vi "connectAndReceiveMessages.vi"(8 "error in (no error)":errorcluster, 9 "remote port":u16, 10 "remote address":string, 11 "NetworkServer in":refnum<class "NetworkServer.lvclass">) -> (0 "error out":errorcluster, 3 "NetworkServer out":refnum<class "NetworkServer.lvclass">)   [LabVIEW 2009, in "Hardware.lvlib" / "HWControllers.lvlib" / "NetworkServer.lvclass"]
uses:
  NetworkServer.lvclass
panel:
  in  "stop":bool
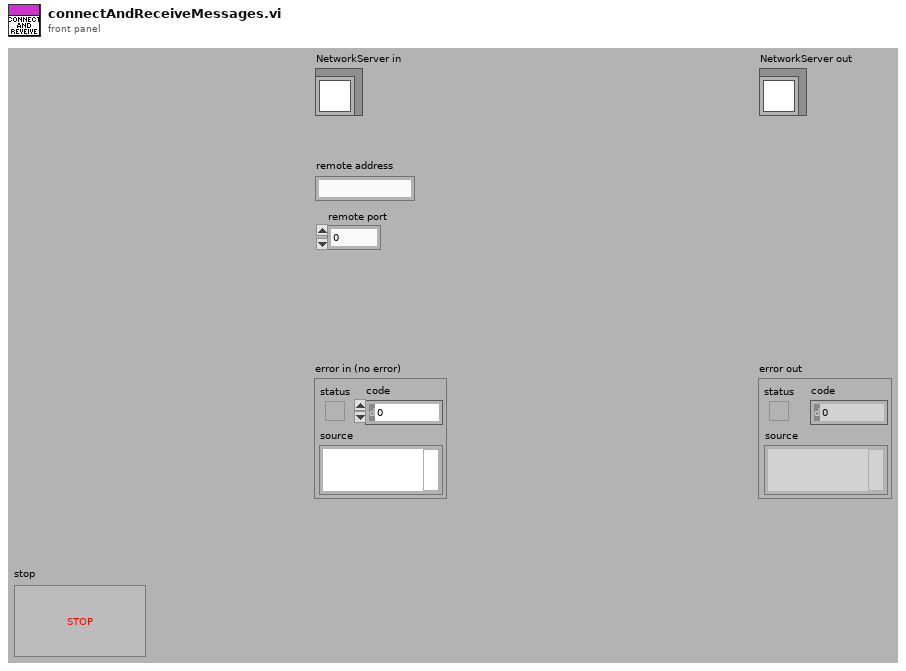
[diagram p1: front panel]
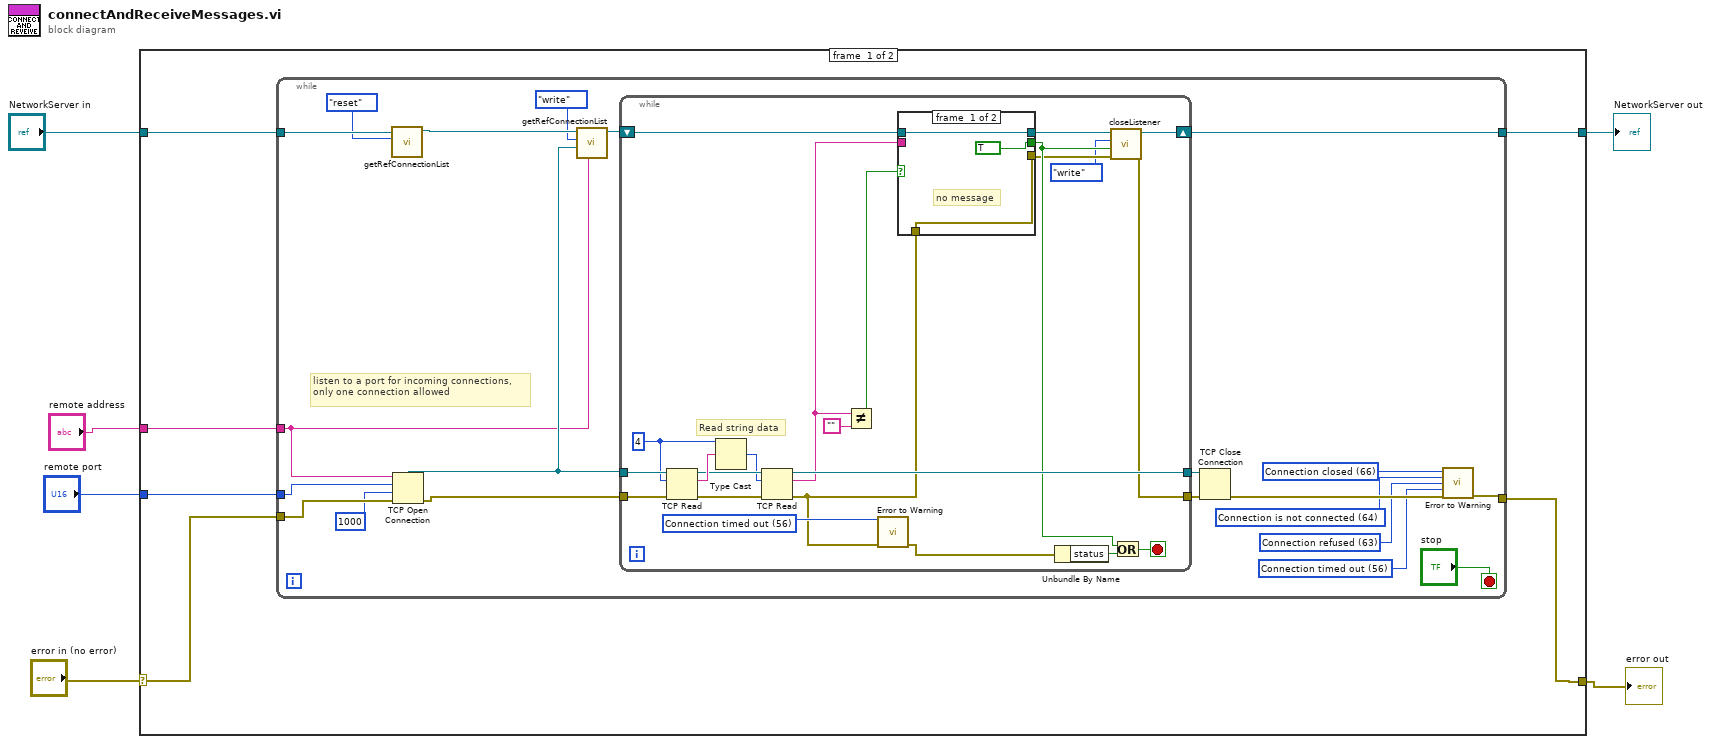
[diagram p0: block diagram]
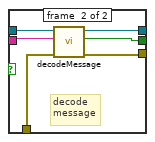
[diagram p2: hidden frame]
diagram:
  n1 = case shown="No Error" "error in (no error)" {
    selector: "error in (no error)" -> [w7 w67]
    tunnel: [w10 w67] -> w4
    tunnel: [w12 w66] -> w5
    tunnel: "NetworkServer in" -> [w11 w66]
    tunnel: "remote address" -> [w9 _]
    tunnel: "remote port" -> [w8 _]
    frame #0 {
      n2 = while {
        tunnel: [w29] -> w12
        tunnel: w11 -> [w19]
        tunnel: [w26] -> w10
        tunnel: w9 -> [w13]
        tunnel: w8 -> [w23]
        tunnel: w7 -> [w22]
        stop <- "stop" stop-if-true
        w20 = 56 items=["No Error", "Argument Error", "Memory Full", "Out of Zone", "End of File", "File Already Open", "Generic File IO Error", "File Not Found", "File Permission Error", "Disk Full", "Duplicate Path", "Too Many Files Open", "Not Enabled", "Resource File Not Found", "Cannot Add Resource", "Resource Not Found", "Image Not Found", "Image Memory Error", "Pen Does Not Exist", "Config Bad Type", "Config Token Not Found", "Config Parse Error", "Config Memory Error", "Bad External Code Format", "Bad External Code Offset", "External Code Not Present", "Null Window", "Destroy Window Mixup", "Null Menu", "Print Aborted", "Bad Print Record", "Print Driver Error", "Windows Error During Print", "Memory Error During Print", "Print Dialog Error", "Generic Print Error", "Invalid Device Refnum", "Device Not Found", "Device Parameter Error", "Device Unit Error", "Can't Open Device", "Device Call Aborted", "Generic Error", "Cancelled By User", "Object ID Too Low", "Object ID Too High", "Object Not In Heap", "Unknown Heap", "Bad DefProc ID", "DefProc Not In Table", "Message Out Of Range", "Null Method", "Unknown Message", "Manager Call Not Supported", "Bad address", "Connection In progress", "Connection timed out", "Connection is already in progress", "Network attribute not supported", "Network error", "Address in use", "System out of memory", "Connection aborted", "Connection refused", "Connection is not connected", "Connection is already connected", "Connection closed", "Initialize error (interapplication manager)", "Bad occurrence", "Wait on unbound occurrence handler", "Occurrence queue overflow", "Bad path", "Semaphore not signaled", "Unrecognized type (interapplication manager)"] ("1st Error to Convert")
        w27 = 63 items=["No Error", "Argument Error", "Memory Full", "Out of Zone", "End of File", "File Already Open", "Generic File IO Error", "File Not Found", "File Permission Error", "Disk Full", "Duplicate Path", "Too Many Files Open", "Not Enabled", "Resource File Not Found", "Cannot Add Resource", "Resource Not Found", "Image Not Found", "Image Memory Error", "Pen Does Not Exist", "Config Bad Type", "Config Token Not Found", "Config Parse Error", "Config Memory Error", "Bad External Code Format", "Bad External Code Offset", "External Code Not Present", "Null Window", "Destroy Window Mixup", "Null Menu", "Print Aborted", "Bad Print Record", "Print Driver Error", "Windows Error During Print", "Memory Error During Print", "Print Dialog Error", "Generic Print Error", "Invalid Device Refnum", "Device Not Found", "Device Parameter Error", "Device Unit Error", "Can't Open Device", "Device Call Aborted", "Generic Error", "Cancelled By User", "Object ID Too Low", "Object ID Too High", "Object Not In Heap", "Unknown Heap", "Bad DefProc ID", "DefProc Not In Table", "Message Out Of Range", "Null Method", "Unknown Message", "Manager Call Not Supported", "Bad address", "Connection In progress", "Connection timed out", "Connection is already in progress", "Network attribute not supported", "Network error", "Address in use", "System out of memory", "Connection aborted", "Connection refused", "Connection is not connected", "Connection is already connected", "Connection closed", "Initialize error (interapplication manager)", "Bad occurrence", "Wait on unbound occurrence handler", "Occurrence queue overflow", "Bad path", "Semaphore not signaled", "Unrecognized type (interapplication manager)"] ("1st Error to Convert")
        w28 = 64 items=["No Error", "Argument Error", "Memory Full", "Out of Zone", "End of File", "File Already Open", "Generic File IO Error", "File Not Found", "File Permission Error", "Disk Full", "Duplicate Path", "Too Many Files Open", "Not Enabled", "Resource File Not Found", "Cannot Add Resource", "Resource Not Found", "Image Not Found", "Image Memory Error", "Pen Does Not Exist", "Config Bad Type", "Config Token Not Found", "Config Parse Error", "Config Memory Error", "Bad External Code Format", "Bad External Code Offset", "External Code Not Present", "Null Window", "Destroy Window Mixup", "Null Menu", "Print Aborted", "Bad Print Record", "Print Driver Error", "Windows Error During Print", "Memory Error During Print", "Print Dialog Error", "Generic Print Error", "Invalid Device Refnum", "Device Not Found", "Device Parameter Error", "Device Unit Error", "Can't Open Device", "Device Call Aborted", "Generic Error", "Cancelled By User", "Object ID Too Low", "Object ID Too High", "Object Not In Heap", "Unknown Heap", "Bad DefProc ID", "DefProc Not In Table", "Message Out Of Range", "Null Method", "Unknown Message", "Manager Call Not Supported", "Bad address", "Connection In progress", "Connection timed out", "Connection is already in progress", "Network attribute not supported", "Network error", "Address in use", "System out of memory", "Connection aborted", "Connection refused", "Connection is not connected", "Connection is already connected", "Connection closed", "Initialize error (interapplication manager)", "Bad occurrence", "Wait on unbound occurrence handler", "Occurrence queue overflow", "Bad path", "Semaphore not signaled", "Unrecognized type (interapplication manager)"] ("1st Error to Convert")
        w32 = 66 items=["No Error", "Argument Error", "Memory Full", "Out of Zone", "End of File", "File Already Open", "Generic File IO Error", "File Not Found", "File Permission Error", "Disk Full", "Duplicate Path", "Too Many Files Open", "Not Enabled", "Resource File Not Found", "Cannot Add Resource", "Resource Not Found", "Image Not Found", "Image Memory Error", "Pen Does Not Exist", "Config Bad Type", "Config Token Not Found", "Config Parse Error", "Config Memory Error", "Bad External Code Format", "Bad External Code Offset", "External Code Not Present", "Null Window", "Destroy Window Mixup", "Null Menu", "Print Aborted", "Bad Print Record", "Print Driver Error", "Windows Error During Print", "Memory Error During Print", "Print Dialog Error", "Generic Print Error", "Invalid Device Refnum", "Device Not Found", "Device Parameter Error", "Device Unit Error", "Can't Open Device", "Device Call Aborted", "Generic Error", "Cancelled By User", "Object ID Too Low", "Object ID Too High", "Object Not In Heap", "Unknown Heap", "Bad DefProc ID", "DefProc Not In Table", "Message Out Of Range", "Null Method", "Unknown Message", "Manager Call Not Supported", "Bad address", "Connection In progress", "Connection timed out", "Connection is already in progress", "Network attribute not supported", "Network error", "Address in use", "System out of memory", "Connection aborted", "Connection refused", "Connection is not connected", "Connection is already connected", "Connection closed", "Initialize error (interapplication manager)", "Bad occurrence", "Wait on unbound occurrence handler", "Occurrence queue overflow", "Bad path", "Semaphore not signaled", "Unrecognized type (interapplication manager)"] ("1st Error to Convert")
        # "listen to a port for incoming connections,\nonly one connection allowed"
        n3 = call "getRefConnectionList.vi"("Enum"=enum16{"read", "write", "reset"}."reset", "NetworkServer in"=w19) -> ("NetworkServer out"=w16:refnum<class "NetworkServer.lvclass">)  [unwired: 5 in, 4 out]
        n4 = TCP Open Connection(address=w13, remote port or service name=w23, timeout ms (60000)=1000, error in (no error)=w22) -> (connection ID=w14:refnum<k5>, error out=w24:errorcluster)  [unwired: 1 in]
        n5 = call "getRefConnectionList.vi"("Remote Connection"=w13, "new client"=w14, "Enum"=enum16{"read", "write", "reset"}."write", "NetworkServer in"=w16) -> ("NetworkServer out"=w17:refnum<class "NetworkServer.lvclass">)  [unwired: 3 in, 4 out]
        n6 = while {
          tunnel: [w51] -> w31
          tunnel: w24 -> [w55]
          tunnel: w14 -> [w56]
          tunnel: [w35] -> w30
          shift-right: [w38] -> w29
          shift-left: w17 -> [w45]
          stop <- w50 stop-if-true
          w42 = 56 items=["No Error", "Argument Error", "Memory Full", "Out of Zone", "End of File", "File Already Open", "Generic File IO Error", "File Not Found", "File Permission Error", "Disk Full", "Duplicate Path", "Too Many Files Open", "Not Enabled", "Resource File Not Found", "Cannot Add Resource", "Resource Not Found", "Image Not Found", "Image Memory Error", "Pen Does Not Exist", "Config Bad Type", "Config Token Not Found", "Config Parse Error", "Config Memory Error", "Bad External Code Format", "Bad External Code Offset", "External Code Not Present", "Null Window", "Destroy Window Mixup", "Null Menu", "Print Aborted", "Bad Print Record", "Print Driver Error", "Windows Error During Print", "Memory Error During Print", "Print Dialog Error", "Generic Print Error", "Invalid Device Refnum", "Device Not Found", "Device Parameter Error", "Device Unit Error", "Can't Open Device", "Device Call Aborted", "Generic Error", "Cancelled By User", "Object ID Too Low", "Object ID Too High", "Object Not In Heap", "Unknown Heap", "Bad DefProc ID", "DefProc Not In Table", "Message Out Of Range", "Null Method", "Unknown Message", "Manager Call Not Supported", "Bad address", "Connection In progress", "Connection timed out", "Connection is already in progress", "Network attribute not supported", "Network error", "Address in use", "System out of memory", "Connection aborted", "Connection refused", "Connection is not connected", "Connection is already connected", "Connection closed", "Initialize error (interapplication manager)", "Bad occurrence", "Wait on unbound occurrence handler", "Occurrence queue overflow", "Bad path", "Semaphore not signaled", "Unrecognized type (interapplication manager)"] ("1st Error to Convert")
          w48 = 4
          # "Read string data"
          n7 = TCP Read(connection ID=w56, bytes to read=w48, error in (no error)=w55) -> (connection ID out=w52:refnum<k5>, data out=w54:string, error out=w53:errorcluster)  [unwired: 1 in, 1 out]
          n8 = Type Cast(type=w48, x=w54) -> (*(type *) &x=w47:i32)
          n9 = TCP Read(connection ID=w52, bytes to read=w47, error in (no error)=w53) -> (connection ID out=w51:refnum<k5>, data out=w43:string, error out=w41:errorcluster)  [unwired: 1 in, 1 out]
          n10 = Not Equal?(x=w43, y="") -> (x != y?=w44:bool)
          n11 = call <vilib>:"Error to Warning.vi"("1st Error to Convert"=w42, "error in"=w41) -> ("warning out"=w40:errorcluster)  [unwired: 3 in, 10 out]
          n12 = case shown="True" w44 {
            tunnel: w45 -> [w59 w65]
            tunnel: [w59 w64] -> w39
            tunnel: w41 -> [w58 w63]
            tunnel: [w58 w62] -> w36
            tunnel: w43 -> [_ w61]
            tunnel: [TRUE w60] -> w37
            frame #0 {
              # "no message"
            }
            frame #1 {
              # "decode\nmessage"
              n13 = call-dynamic "decodeMessage.vi"("error in (no error)"=w63, "MessageString"=w61, "NetworkClient in"=w65) -> ("error out"=w62:errorcluster, "close"=w60:bool, "NetworkClient out"=w64:refnum<class "NetworkServer.lvclass">)  [unwired: 6 in]
            }
          }
          n14 = Unbundle By Name(w40) -> ("status"=w49:bool)
          n15 = call "closeListener.vi"("error in (no error)"=w36, "close"=w37, "actions"=enum16{"read", "write"}."write", "NetworkServer in"=w39) -> ("error out"=w35:errorcluster, "NetworkServer out"=w38:refnum<class "NetworkServer.lvclass">)  [unwired: 5 in, 1 out]
          n16 = Or(x=w37, y=w49) -> (x .or. y?=w50:bool)
        }
        n17 = TCP Close Connection(connection ID=w31, error in (no error)=w30) -> (error out=w33:errorcluster)  [unwired: 1 in, 1 out]
        n18 = call <vilib>:"Error to Warning.vi"("1st Error to Convert"=w32, "2nd Error to Convert"=w28, "3rd Error to Convert"=w27, "4th Error to Convert"=w20, "error in"=w33) -> ("warning out"=w26:errorcluster)  [unwired: 10 out]
      }
    }
    frame #1 {
    }
  }
  "error out" <- w4
  "NetworkServer out" <- w5
